vi "Tektronix AFG 3000 Series Generate Arbitrary Waveform.vi"() -> ()   [LabVIEW 2015]
doc: "Demonstrates how to configure then create an arbitrary waveform."
uses:
  Instance           2 61Saved   Tektronix AFG 3000 Series Generate Arbitrary Waveform .vi
  Instance           1 61Saved   Tektronix AFG 3000 Series Generate Arbitrary Waveform .vi
  Tektronix AFG 3000 Series.lvlib
panel:
  in  "Frequency (1000 Hz)":dbl=1000.0
  in  "DC Offset (0 V)":dbl
  in  "Gain (1 V)":dbl=1.0
  in  "Arbitrary Waveform Name (0: USER1)":u16(ring) items=["USER1", "USER2", "USER3", "USER4"]
  in  "Channel (0: Channel 1)":u16(ring) items=["Channel 1", "Channel 2"]
  in  "VISA resource name":refnum<visa-resource-name>
  # "(c) 2006-2013 National Instruments.  ALL RIGHTS RESERVED."
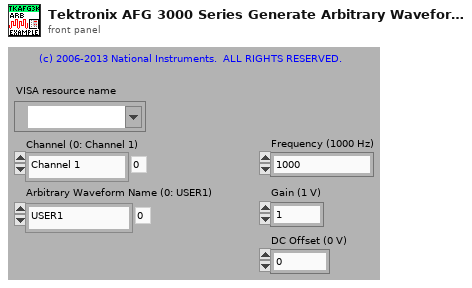
[diagram p1: front panel]
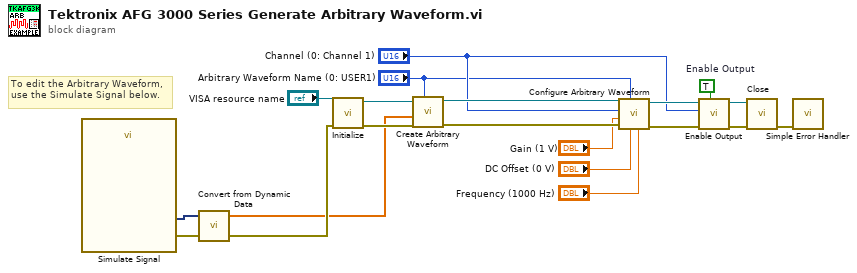
[diagram p0: block diagram]
diagram:
  w9 = TRUE  # Enable Output
  # "To edit the Arbitrary Waveform, use the Simulate Signal below."
  n1 = call "Simulate Signal"() -> ("Sine with Uniform Noise"=w2:dynamicdata, "error out"=w11:errorcluster)  [unwired: 14 in]
  n2 = call "Convert from Dynamic Data"("Dynamic Data Type"=w2) -> ("Array"=w1:dbl[])  [unwired: 3 in]
  n3 = call "Initialize.vi"("error in (no error)"=w11, "VISA resource name"="VISA resource name") -> ("error out"=w12:errorcluster, "VISA resource name out"=w8:refnum<visa-resource-name>)  [unwired: 8 in]
  n4 = call "Create Arbitrary Waveform.vi"("Arbitrary Waveform Name (0: USER1)"="Arbitrary Waveform Name (0: USER1)", "error in (no error)"=w12, "Arbitrary Waveform Data"=w1, "VISA resource name"=w8) -> ("error out"=w14:errorcluster, "VISA resource name out"=w15:refnum<visa-resource-name>)  [unwired: 6 in]
  n5 = call "Configure Arbitrary Waveform.vi"("Frequency (1000 Hz)"="Frequency (1000 Hz)", "DC Offset (0 V)"="DC Offset (0 V)", "Arbitrary Waveform Name (0: USER1)"="Arbitrary Waveform Name (0: USER1)", "error in (no error)"=w14, "Gain (1 V)"="Gain (1 V)", "Channel (0: Channel 1)"="Channel (0: Channel 1)", "VISA resource name"=w15) -> ("error out"=w13:errorcluster, "VISA resource name out"=w16:refnum<visa-resource-name>)  [unwired: 3 in]
  n6 = call "Enable Output.vi"("Enable Output (T: Enable)"=w9, "error in (no error)"=w13, "Channel (0: Channel 1)"="Channel (0: Channel 1)", "VISA resource name"=w16) -> ("error out"=w17:errorcluster, "VISA resource name out"=w18:refnum<visa-resource-name>)  [unwired: 6 in]
  n7 = call "Close.vi"("error in (no error)"=w17, "VISA resource name"=w18) -> ("error out"=w19:errorcluster)  [unwired: 9 in]
  n8 = call <vilib>:"Simple Error Handler.vi"("error in (no error)"=w19) -> ()  [unwired: 4 in, 5 out]
